vi "Obtain Notifier.vi"(8 "error in":errorcluster) -> (0 "error out":errorcluster, 3 "Notifier Out":T1)   [LabVIEW 2022 SP3]
uses:
  Controls/Notifier ctl.ctl
  Controls/Notifier data ctl.ctl
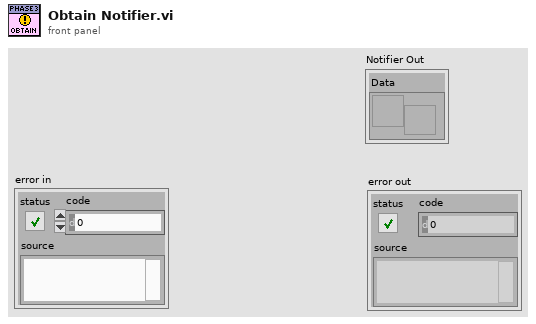
[diagram p1: front panel]
types:
  T1 = typedef "Notifier ctl.ctl" = cluster{"Data":refnum<notifier>}
  T2 = typedef "Notifier data ctl.ctl" = cluster{"Message":string, "Data":variant}
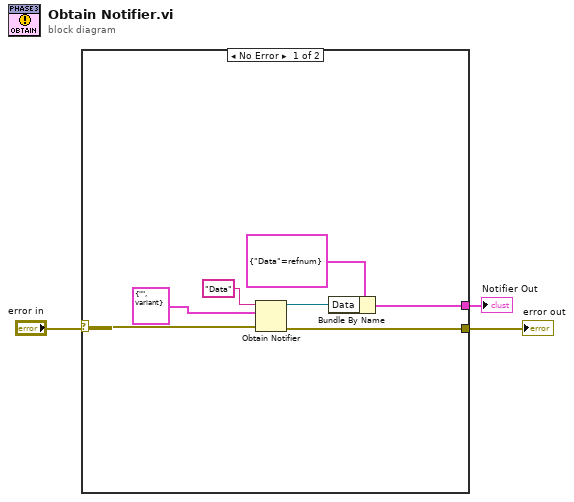
[diagram p0: block diagram]
diagram:
  n1 = case shown="No Error" "error in" {
    selector: "error in" -> [w10 w11]
    tunnel: [w8 w11] -> w2
    tunnel: [w4 _] -> w1
    frame No Error {
      n2 = Obtain Notifier(name (unnamed)="Data", notification data type=T2 {"Message"="", "Data"=variant(digitalwaveform[] [])}, error in (no error)=w10) -> (notifier out=w5:refnum<notifier>, error out=w8:errorcluster)  [unwired: 1 in, 1 out]
      n3 = Bundle By Name(cluster=T1 {"Data"=refnum} ("Cluster"), "Data"=w5) -> (w4:T1)
    }
    frame Error {
    }
  }
  "error out" <- w2
  "Notifier Out" <- w1
